vi "UDP Server Gyro.vi"(8 "error in (no error)":errorcluster, 10 "User Event in":refnum<class "User Event.lvclass">, 11 "UDP Port":u16=5015) -> (0 "error out":errorcluster)   [LabVIEW 2016]
uses:
  User Events/User Event.lvclass
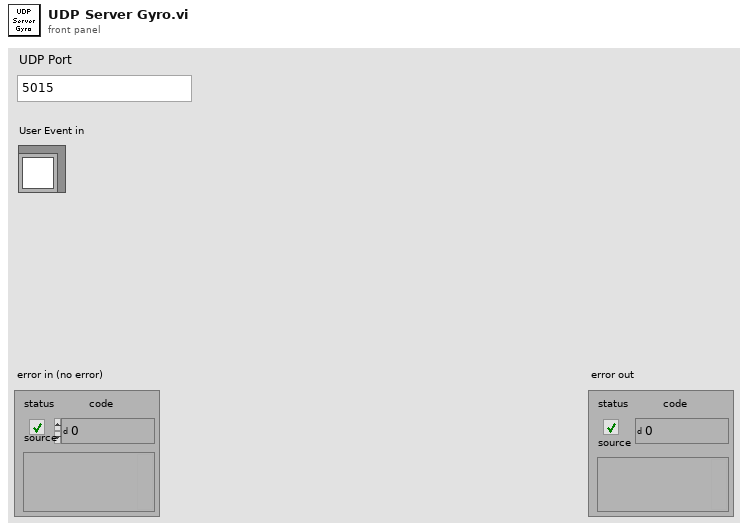
[diagram p1: front panel]
types:
  T1 = typedef "M1M3SupSimUserEvents.ctl" = cluster{"ILCResponse":refnum<user-event>, "StopUDPServer":refnum<user-event>, "InclinometerResponse":refnum<user-event>, "DisplaceResponse":refnum<user-event>, "AccelerometerResponse":refnum<user-event>, "DigitalInput":refnum<user-event>, "DigitalOutput":refnum<user-event>, "GyroResponse":refnum<user-event>}
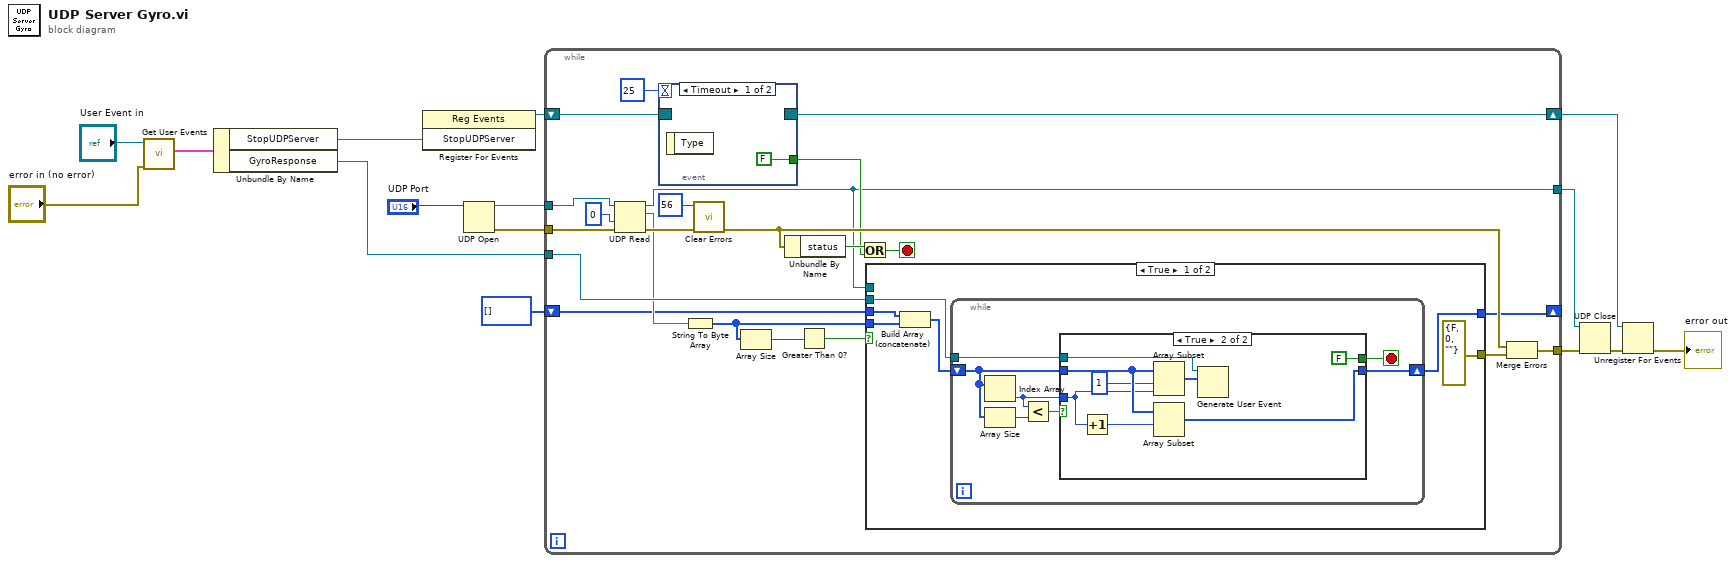
[diagram p0: block diagram]
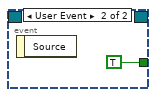
[diagram p2: hidden frame]
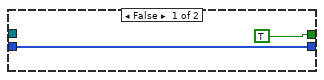
[diagram p3: hidden frame]
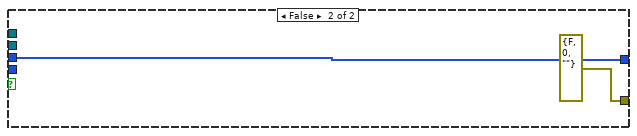
[diagram p4: hidden frame]
diagram:
  n1 = call "Get User Events.vi"("error in (no error)"="error in (no error)", "User Event in"="User Event in") -> ("User Events"=w15:T1)  [unwired: 7 in, 2 out]
  n2 = Unbundle By Name(w15) -> ("StopUDPServer"=w4:refnum<user-event>, "GyroResponse"=w3:refnum<user-event>)
  n3 = register-events(w4) -> (reference out=w7:refnum<event-registration>)  [unwired: 2 in, 1 out]
  n4 = UDP Open(11:"UDP Port") -> (port=w11:refnum<k16>, 0:w10:errorcluster)  [unwired: 4 in, 1 out]
  n5 = while {
    tunnel: w11 -> [w37]
    tunnel: w10 -> [w36]
    tunnel: [w29] -> w8
    tunnel: [w22] -> w9
    shift-right: [w24] -> w5
    shift-left: w7 -> [w27]
    tunnel: w3 -> [w23]
    shift-right: [w19] -> _
    shift-left: u8[] [] ("unsigned byte array") -> [w20]
    stop <- w28 stop-if-true
    n6 = UDP Read(connection ID=w37, timeout ms (25000)=0, 8:w36) -> (data out=w21:string, error out=w34:errorcluster, 3:w22:refnum<k16>)  [unwired: 1 in, 2 out]
    n7 = event shown="[0] Timeout" {
      selector: w27 -> [_ _]
      dyn-events: [_ _] -> w24
      timeout: 25 -> [_ _]
      tunnel: [FALSE TRUE] -> w25
      event Timeout {
        n8 = event-data() -> ()  [unwired: 1 in, 1 out]
      }
      event User Event {
        n9 = event-data() -> ()  [unwired: 1 in, 1 out]
      }
    }
    n10 = String To Byte Array(string=w21) -> (unsigned byte array=w18:u8[])
    n11 = call <vilib>:"Clear Errors.vi"("error in (no error)"=w34, "specific error code to clear (0: all)"=56) -> ("error out"=w31:errorcluster)  [unwired: 4 in, 1 out]
    n12 = Array Size(array=w18) -> (size(s)=w17:i32)
    n13 = Unbundle By Name(w31) -> ("status"=w32:bool)
    n14 = Greater Than 0?(x=w17) -> (x > 0?=w16:bool)
    n15 = Or(x=w32, y=w25) -> (x .or. y?=w28:bool)
    n16 = case shown="True" w16 {
      tunnel: [errorcluster {"status"=FALSE, "code"=0, "source"=""} ("error out") errorcluster {"status"=FALSE, "code"=0, "source"=""} ("error out")] -> w30
      tunnel: w23 -> [w42 _]
      tunnel: w22 -> [_ _]
      tunnel: w18 -> [w44 _]
      tunnel: w20 -> [w45 w63]
      tunnel: [w40 w63] -> w19
      frame True {
        n17 = Build Array (concatenate)(w45, w44) -> (w43:u8[])
        n18 = while {
          tunnel: w42 -> [w51]
          shift-right: [w49] -> w40
          shift-left: w43 -> [w48]
          stop <- w50 stop-if-true
          n19 = Index Array(array=w48) -> (element=w46:u8)  [unwired: 1 in]
          n20 = Array Size(array=w48) -> (size(s)=w47:i32)
          n21 = Less?(x=w46, y=w47) -> (x < y?=w52:bool)
          n22 = case shown="True" w52 {
            tunnel: w48 -> [w54 w60]
            tunnel: w46 -> [_ w55]
            tunnel: w51 -> [_ w61]
            tunnel: [w54 w59] -> w49
            tunnel: [TRUE FALSE] -> w50
            frame False {
            }
            frame True {
              n23 = Increment(x=w55) -> (x+1=w56:u8)
              n24 = Array Subset(array=w60, index=1, length=w55) -> (w62:u8[])
              n25 = Array Subset(array=w60, index=w56) -> (w59:u8[])  [unwired: 1 in]
              n26 = Generate User Event(user event=w61, event data cluster=w62) -> ()  [unwired: 2 in, 2 out]
            }
          }
        }
      }
      frame False {
      }
    }
    n27 = Merge Errors(w31, w30) -> (w29:errorcluster)
  }
  n28 = UDP Close(connection ID=w9, 8:w8) -> (error out=w6:errorcluster)  [unwired: 1 out]
  n29 = Unregister For Events(event registration refnum=w5, error in=w6) -> (error out=→"error out":errorcluster)
